vi "unsubscribe in mapping.vi"(6 "publishing module ID":string, 7 "subscribing module ID":string, 8 "error in":errorcluster, 9 "published element":string, 10 "subscribed element":string, 11 "mappings in":T1) -> (0 "error out":errorcluster, 3 "mappings out":T1)   [LabVIEW 2013, in "engine configuration.lvclass"]
uses:
  engine configuration.lvclass
  simple mapping.ctl
  module channel pairings.ctl
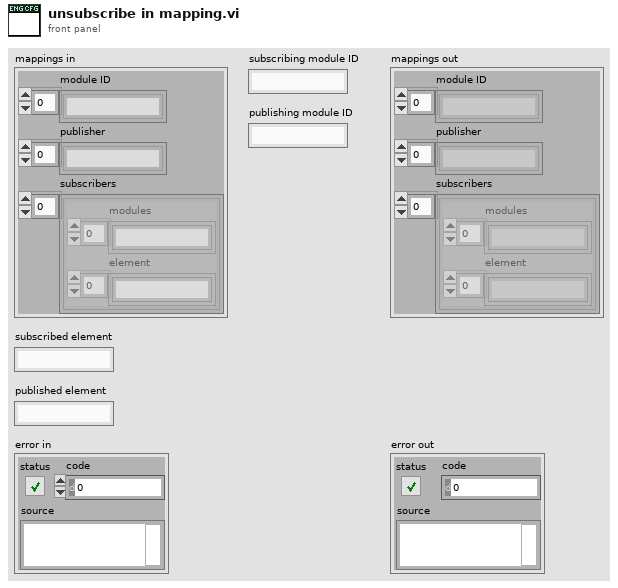
[diagram p1: front panel]
types:
  T1 = typedef "engine configuration.lvclass/simple mapping.ctl" = cluster{"module ID":string[], "publisher":string[], "subscribers":T2[]}
  T2 = typedef "engine configuration.lvclass/module channel pairings.ctl" = cluster{"modules":string[], "element":string[]}
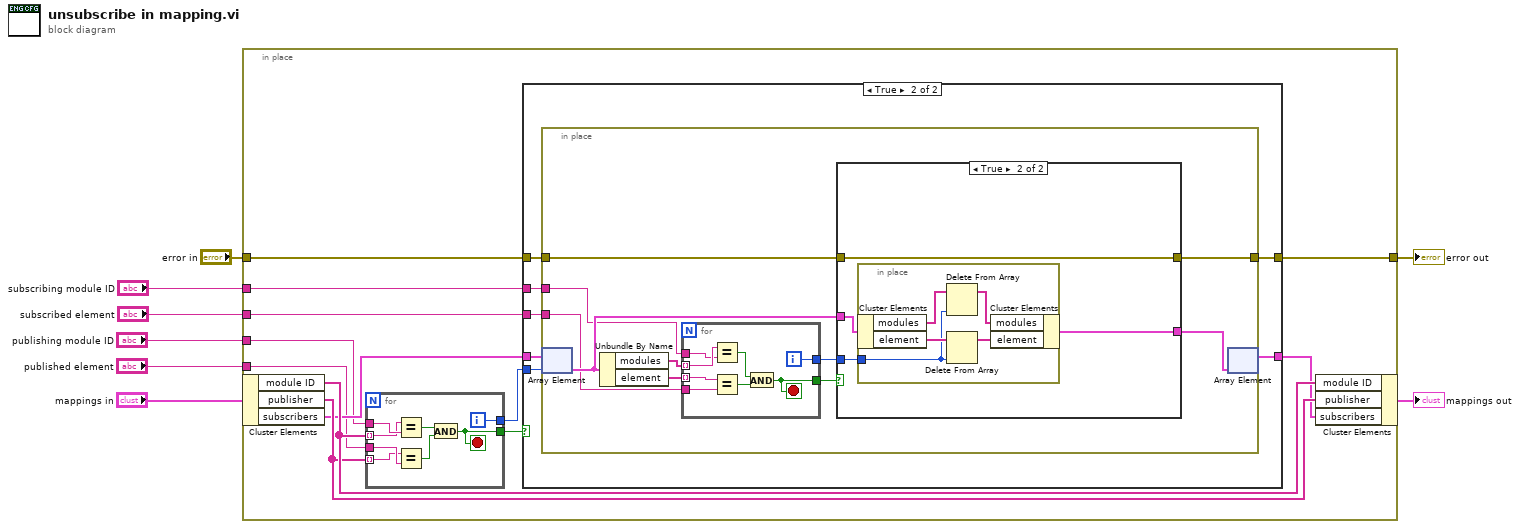
[diagram p0: block diagram]
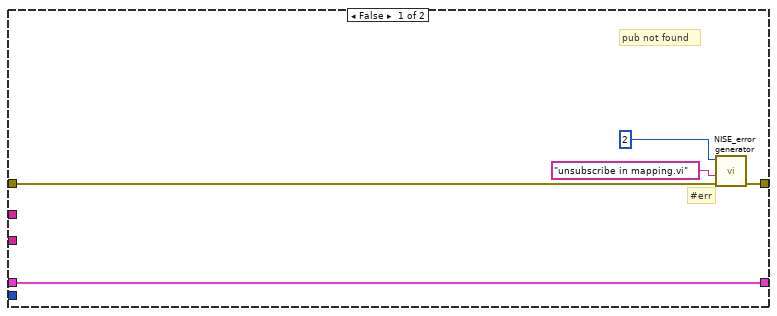
[diagram p2: hidden frame]
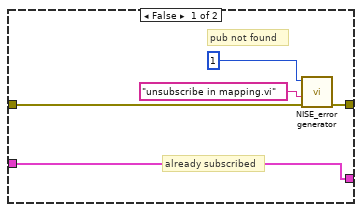
[diagram p3: hidden frame]
diagram:
  n1 = in-place {
    in-place-border: "subscribing module ID" -> [w14]
    in-place-border: "subscribed element" -> [w13]
    in-place-border: [w16] -> w7
    in-place-border: "error in" -> [w15]
    in-place-border: "publishing module ID" -> [w12]
    in-place-border: "published element" -> [w11]
    n2 = in-place-cluster #1("mappings in") -> ("module ID"=w20:string[], "publisher"=w19:string[], "subscribers"=w17:T2[])
    n3 = for {
      tunnel: [w26] -> w10
      tunnel: w12 -> [w25]
      tunnel: w11 -> [w24]
      tunnel: w20 -> [w23] mode=indexing
      tunnel: w19 -> [w22] mode=indexing
      tunnel: [w21] -> w9
      i -> [w21]
      stop <- w26 stop-if-true
      n4 = Equal?(x=w23, y=w25) -> (x = y?=w27:bool)
      n5 = Equal?(x=w22, y=w24) -> (x = y?=w28:bool)
      n6 = And(x=w27, y=w28) -> (x .and. y?=w26:bool)
    }
    n7 = case shown="True" w10 {
      tunnel: [w32 w35] -> w16
      tunnel: w15 -> [w33 w34]
      tunnel: [w29 w38] -> w18
      tunnel: w17 -> [w29 w39]
      tunnel: w14 -> [_ w36]
      tunnel: w13 -> [_ w37]
      tunnel: w9 -> [_ w40]
      frame False {
        # "pub not found"
        # "#err"
        n8 = call <vilib>:"NISE_error generator.vi"("error in"=w33, "source"="unsubscribe in mapping.vi", "error code (0)"=2) -> ("error out"=w32:errorcluster)  [unwired: 6 in]
      }
      frame True {
        n9 = in-place {
          in-place-border: w37 -> [w45]
          in-place-border: w36 -> [w44]
          in-place-border: [w43] -> w35
          in-place-border: w34 -> [w42]
          n10 = in-place-array #2(w39, w40) -> (w47:T2)
          n11 = Unbundle By Name(w47) -> ("modules"=w50:string[], "element"=w49:string[])
          n12 = for {
            tunnel: w50 -> [w70] mode=indexing
            tunnel: w49 -> [w69] mode=indexing
            tunnel: w45 -> [w68]
            tunnel: w44 -> [w67]
            tunnel: [w66] -> w48
            tunnel: [w65] -> w41
            i -> [w65]
            stop <- w66 stop-if-true
            n13 = Equal?(x=w70, y=w67) -> (x = y?=w72:bool)
            n14 = Equal?(x=w69, y=w68) -> (x = y?=w71:bool)
            n15 = And(x=w72, y=w71) -> (x .and. y?=w66:bool)
          }
          n16 = case shown="True" w48 {
            tunnel: w47 -> [w55 w59]
            tunnel: [w55 w58] -> w46
            tunnel: [w51 w57] -> w43
            tunnel: w42 -> [w52 w57]
            tunnel: w41 -> [_ w56]
            frame False {
              # "pub not found"
              # "already subscribed"
              n17 = call <vilib>:"NISE_error generator.vi"("error in"=w52, "source"="unsubscribe in mapping.vi", "error code (0)"=1) -> ("error out"=w51:errorcluster)  [unwired: 6 in]
            }
            frame True {
              n18 = in-place {
                in-place-border: w56 -> [w60]
                n19 = in-place-cluster #3(w59) -> ("modules"=w63:string[], "element"=w64:string[])
                n20 = Delete From Array(array=w63, index=w60) -> (array with subset deleted=w62:string[])  [unwired: 1 in, 1 out]
                n21 = Delete From Array(array=w64, index=w60) -> (array with subset deleted=w61:string[])  [unwired: 1 in, 1 out]
                n22 = in-place-cluster #3("modules"=w62, "element"=w61) -> (w58:T2)
              }
            }
          }
          n23 = in-place-array #2(w46) -> (w38:T2[])  [unwired: 1 out]
        }
      }
    }
    n24 = in-place-cluster #1("module ID"=w20, "publisher"=w19, "subscribers"=w18) -> (→"mappings out":T1)
  }
  "error out" <- w7
